vi "HowToAdjustAngleTest.vi"() -> (3 "Were there any errors at all?":bool)   [LabVIEW 2013]
uses:
  Data/TypeDefs/Sailing Regimes.ctl
panel:
  in  "Regime inputs":T1[](array[typedef])=[enum."Upwind - Port Tack", enum."Upwind - Starboard Tack", enum."Reach - Port Tack", enum."Run - Starboard Tack", enum."Run - Port Tack", enum."Reach - Port Tack"]
  in  "Expected regime outputs":T1[](array[typedef])=[enum."Upwind - Port Tack", enum."Upwind - Starboard Tack", enum."Reach - Port Tack", enum."Run - Starboard Tack", enum."Run - Port Tack", enum."Reach - Port Tack"]
  out "Actual regime outputs":T1[](array[typedef])=[enum."Upwind - Port Tack", enum."Upwind - Starboard Tack", enum."Reach - Port Tack", enum."Run - Starboard Tack", enum."Run - Port Tack", enum."Reach - Port Tack"]
  out "Are chosen regimes right?":bool[](array[boolean])=[TRUE, TRUE, TRUE, TRUE, TRUE, TRUE]
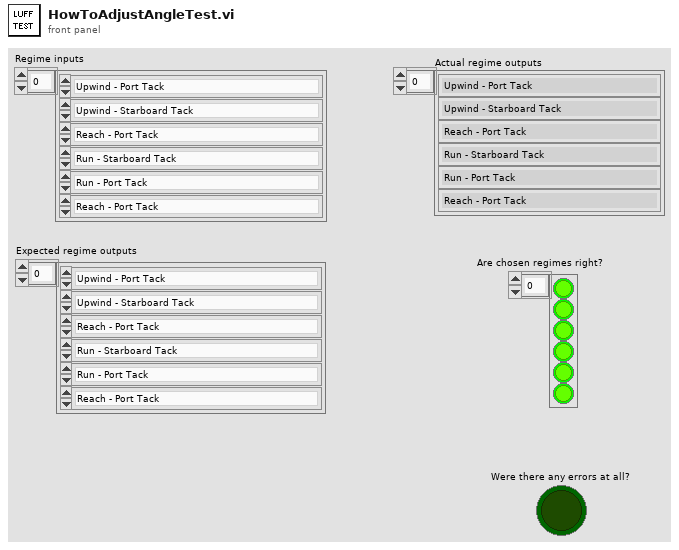
[diagram p1: front panel]
types:
  T1 = typedef "Sailing Regimes.ctl" = enum16{"Tack - Bow across wind", "Upwind - Starboard Tack", "Turn between Upwind/Reach - Starboard Tack", "Reach - Starboard Tack", "Turn between Reach/Run - Starboard Tack", "Run - Starboard Tack", "Jibe - Stern across wind", "Run - Port Tack", "Turn between Reach/Run - Port Tack", "Reach - Port Tack", "Turn between Upwind/Reach - Port Tack", "Upwind - Port Tack"}
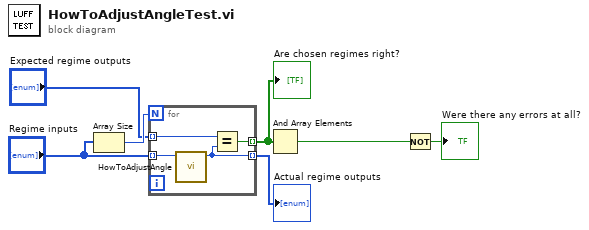
[diagram p0: block diagram]
diagram:
  n1 = Array Size(array="Regime inputs") -> (size(s)=w7:i32)
  n2 = for {
    N: w7 -> [_]
    tunnel: "Expected regime outputs" -> [w11] mode=indexing
    tunnel: [w10] -> w6 mode=indexing
    tunnel: "Regime inputs" -> [w9] mode=indexing
    tunnel: [w8] -> w1 mode=indexing
    n3 = call "HowToAdjustAngle.vi"("Current Sailing Regime"=w9) -> ("Desired Sailing Regime"=w8:T1)  [unwired: 10 in]
    n4 = Equal?(x=w11, y=w8) -> (x = y?=w10:bool)
  }
  "Are chosen regimes right?" <- w6
  "Actual regime outputs" <- w1
  n5 = And Array Elements(Boolean array=w6) -> (logical AND=w4:bool)
  n6 = Not(x=w4) -> (.not. x?=→"Were there any errors at all?":bool)
